vi "AMWave.vi"(9 "AM Wave Parameters":T1={"Signal Frequency "=500.0, "Modulation Frequency"=50.0, "Amplitude"=1.0}, 10 "Digitizing Parameters":T2={"Number of Samples"=500.0, "Sampling Frequency"=10000.0}) -> (2 "AM Wave":cluster{"Time":dbl[], "Displacement":dbl[]})   [LabVIEW 2013]
uses:
  <vilib>/imath/engines/lvmath2/RunTimeEngine/ErrorHandling/NIMS_Finalize Error.vi
  <vilib>/imath/engines/lvmath2/RunTimeEngine/Managers/WorkSpace/UID Generator.vi
  <vilib>/imath/engines/lvmath2/RunTimeEngine/Managers/SymbolTable/Clear UID.vi
  <vilib>/imath/engines/lvmath2/RunTimeEngine/NodeEndStatement/NIMS_NodeEndStatement_Output.vi
  <instcachedir>/0/NIMS_NodeEndStatement_Output_53EC0D466D134D7ABD903AC30B43404B.lvgen/NIMS_NodeEndStatement_Output_53EC0D466D134D7ABD903AC30B43404B_005.vi
  <vilib>/imath/engines/lvmath2/RunTimeEngine/RunTimeType/NIMS_RunTimeType_From StrictType (excl LVString).vi
  <instcachedir>/0/NIMS_RunTimeType_From StrictType (excl LVString)_57CF553C4D5778428DA95AEC531EE8B5.lvgen/NIMS_RunTimeType_From StrictType (excl LVString)_57CF553C4D5778428DA95AEC531EE8B5_000.vi
  <vilib>/imath/engines/lvmath2/RunTimeEngine/LocalVariableDefStatement/MC_LocalVariableDefStatement_Display.vi
  <vilib>/imath/engines/lvmath2/RunTimeEngine/RangeToken/NIMS_Range.vi
  <instcachedir>/0/NIMS_Range_CC84A22A7D615C41BA1124D7A0F122CE.lvgen/NIMS_Range_CC84A22A7D615C41BA1124D7A0F122CE_000.vi
  <vilib>/imathl/engines/lvmath/Functions/Error Handling/Create Error.vi
  <vilib>/imath/engines/lvmath2/RunTimeEngine/ArithmeticOperatorToken/NIMS_ArithmeticOperator_times.vi
  <instcachedir>/0/NIMS_ArithmeticOperator_times_9FAC44C088B07F41B9AEF9D97164B37A.lvgen/NIMS_ArithmeticOperator_times_9FAC44C088B07F41B9AEF9D97164B37A_000.vi
  <vilib>/imath/engines/lvmath2/RunTimeEngine/Managers/SymbolTable/NIMS_WorkSpace.lvlib
panel:
  out "XY Graph":cluster{"t":dbl[], "d":dbl[]}(graph)
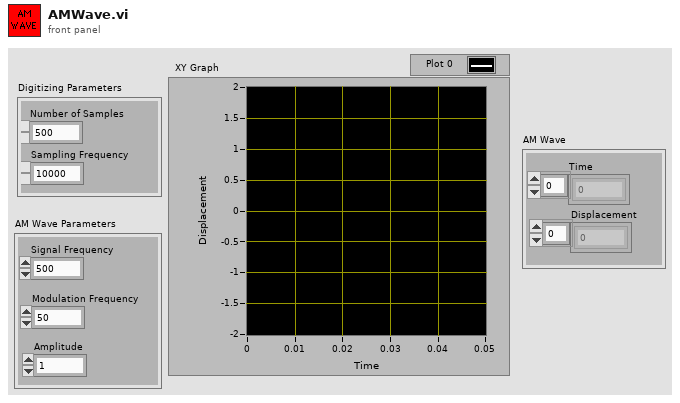
[diagram p1: front panel]
types:
  T1 = cluster{"Signal Frequency ":dbl, "Modulation Frequency":dbl, "Amplitude":dbl}
  T2 = cluster{"Number of Samples":dbl, "Sampling Frequency":dbl}
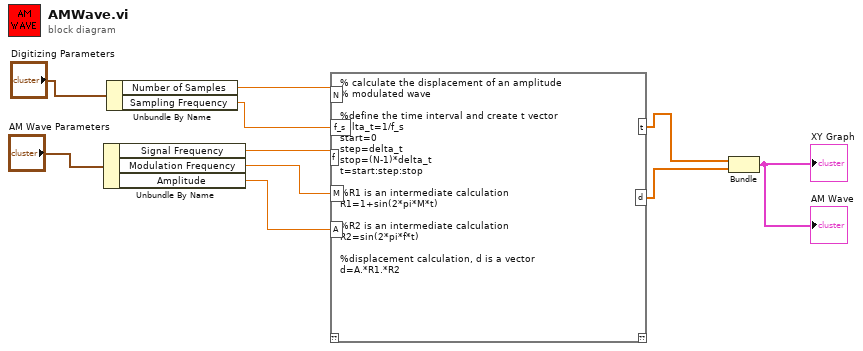
[diagram p0: block diagram]
diagram:
  n1 = Unbundle By Name("AM Wave Parameters") -> ("Signal Frequency"=w6:dbl, "Modulation Frequency"=w5:dbl, "Amplitude"=w4:dbl)
  n2 = Unbundle By Name("Digitizing Parameters") -> ("Number of Samples"=w7:dbl, "Sampling Frequency"=w8:dbl)
  n3 = mathscript code="% calculate the displacement of an amplitude\n% modulated wave\n\n%define the time interval and create t vector\ndelta_t=1/f_s\nstart=0\nstep=delta_t\nstop=(N-1)*delta_t\nt=start:step:stop\n\n%R1 is an intermediate calculation\nR1=1+sin(2*pi*M*t) \n\n%R2 is an intermediate calculation\nR2=sin(2*pi*f*t)\n\n%displacement calculation, d is a vector\nd=A.*R1.*R2"("N"=w7, "f_s"=w8, "f"=w6, "M"=w5, "A"=w4) -> ("t"=w3:dbl[], "d"=w2:dbl[])  [unwired: 1 in, 1 out]
  n4 = Bundle("t"=w3, "d"=w2) -> (→"AM Wave" →"XY Graph":cluster{"t":dbl[], "d":dbl[]})  [unwired: 1 in]
